vi "Clean FreeCache By Name.vi"(8 "error in (no error)":errorcluster, 10 "String":string, 11 "MDPtrMgr in":refnum<class "MDPtrMgr.lvclass">) -> (0 "error out":errorcluster, 3 "MDPtrMgr out":refnum<class "MDPtrMgr.lvclass">)   [LabVIEW 2017, in "MDPtr.lvlib" / "MDPtrMgr.lvclass"]
uses:
  MDPtrMgr.lvclass
  MDPtrMgr.lvclass/MDPtrMgr.ctl
  Factory/Def-MDPtrQ.ctl
  MDPtr TypeDef/MDPtr DataFrame-Memory.ctl
  MDPtr TypeDef/MDPtr DataFrame-Common.ctl
  <vilib>/Utility/Data Type/Type Definitions/Data Type.ctl
  <vilib>/Utility/Data Type/NI_Data Type.lvlib
  MDPtr.lvlib
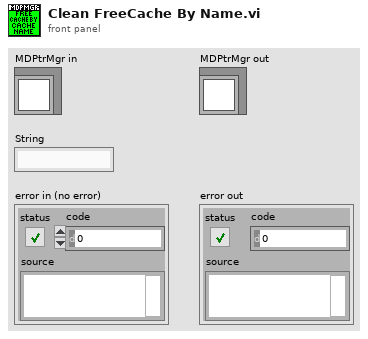
[diagram p1: front panel]
types:
  T1 = typedef "MDPtr.lvlib/MDPtrMgr.lvclass/Def-MDPtrQ.ctl" = refnum<queue>
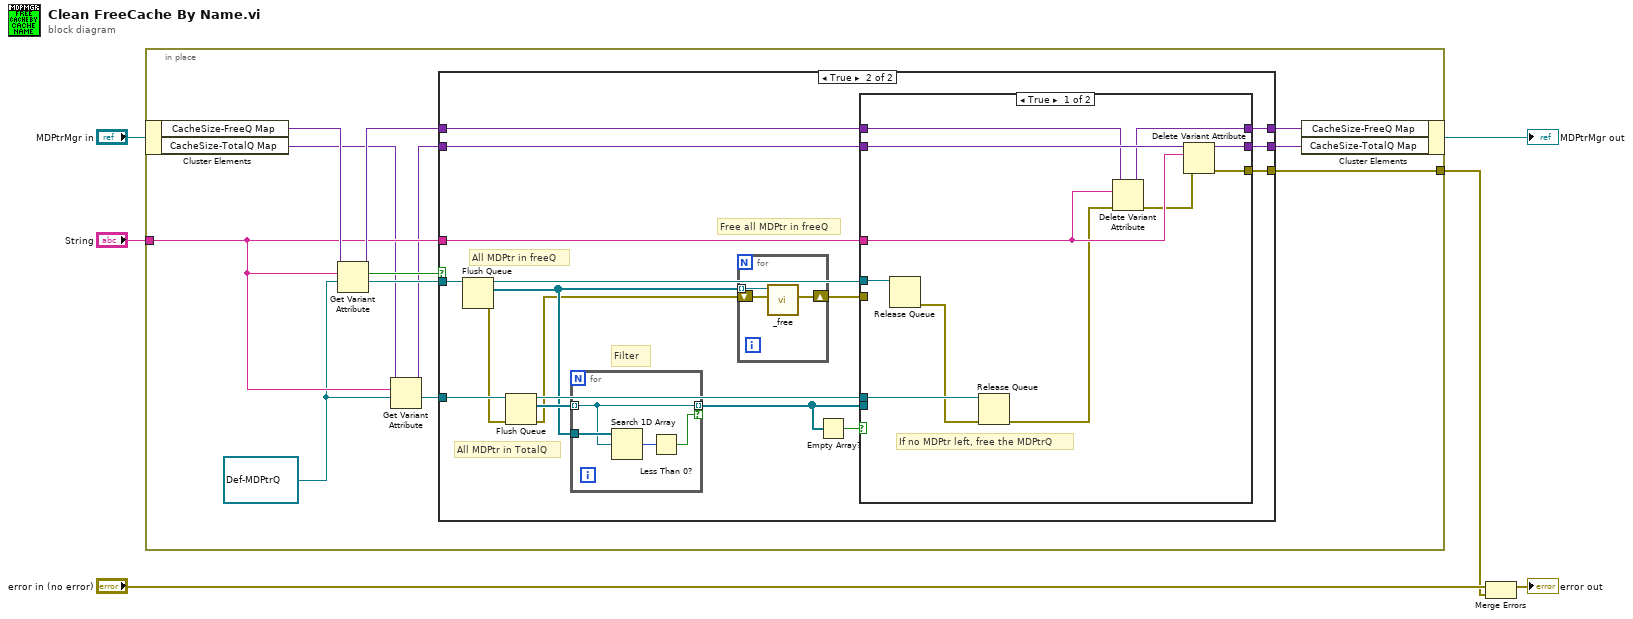
[diagram p0: block diagram]
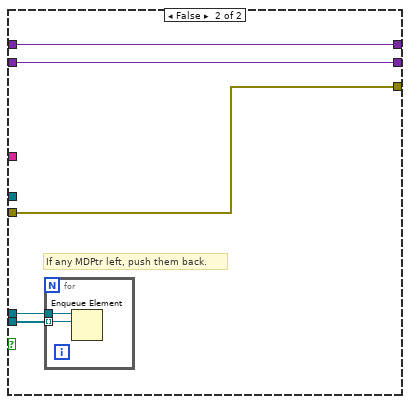
[diagram p3: hidden frame]
diagram:
  n1 = in-place "In Place Element Structure" {
    in-place-border: "String" -> [w12]
    in-place-border: [w7] -> w5
    w11 = T1 refnum ("MDPtrQueue")
    n2 = in-place-cluster #1("MDPtrMgr in") -> ("CacheSize-FreeQ Map"=w18:variant, "CacheSize-TotalQ Map"=w10:variant)
    n3 = Get Variant Attribute(Variant=w18, name=w12, default value (empty Variant)=w11) -> (duplicate Variant=w16:variant, found=w14:bool, value=w13:T1)  [unwired: 1 in, 1 out]
    n4 = Get Variant Attribute(Variant=w10, name=w12, default value (empty Variant)=w11) -> (duplicate Variant=w9:variant, value=w8:T1)  [unwired: 1 in, 2 out]
    n5 = case shown="True" w14 {
      tunnel: [w20 w37] -> w17
      tunnel: w9 -> [w20 w36]
      tunnel: w16 -> [w19 w35]
      tunnel: [w19 w34] -> w15
      tunnel: w12 -> [_ w33]
      tunnel: w13 -> [_ w31]
      tunnel: w8 -> [_ w30]
      tunnel: [_ w32] -> w7
      frame False {
      }
      frame True {
        # "Free all MDPtr in freeQ"
        # "Filter"
        # "All MDPtr in TotalQ"
        # "All MDPtr in freeQ"
        n6 = Flush Queue(queue=w31) -> (queue out=w24:T1, remaining elements=w25:refnum<data-value>[], error out=w23:errorcluster)  [unwired: 1 in]
        n7 = Flush Queue(queue=w30, error in (no error)=w23) -> (queue out=w28:T1, remaining elements=w29:refnum<data-value>[], error out=w22:errorcluster)
        n8 = for {
          tunnel: w29 -> [w60] mode=indexing
          tunnel: w25 -> [w62]
          tunnel: [w60] -> w27 mode=indexing if=w59
          n9 = Search 1D Array(1D array=w62, element=w60) -> (index of element=w61:i32)  [unwired: 1 in]
          n10 = Less Than 0?(x=w61) -> (x < 0?=w59:bool)
        }
        n11 = for {
          tunnel: w25 -> [w40] mode=indexing
          shift-right: [w38] -> w21
          shift-left: w22 -> [w39]
          n12 = call "_free.vi"("error in (no error)"=w39, "MDPtr DVR"=w40) -> ("error out"=w38:errorcluster)  [unwired: 8 in]
        }
        n13 = Empty Array?(array=w27) -> (empty?=w26:bool)
        n14 = case shown="True" w26 {
          tunnel: [w51 w56] -> w37
          tunnel: w36 -> [w50 w56]
          tunnel: w35 -> [w49 w55]
          tunnel: [w48 w55] -> w34
          tunnel: w33 -> [w47 _]
          tunnel: [w45 w52] -> w32
          tunnel: w28 -> [w44 w54]
          tunnel: w27 -> [_ w53]
          tunnel: w24 -> [w43 _]
          tunnel: w21 -> [_ w52]
          frame True {
            # "If no MDPtr left, free the MDPtrQ"
            n15 = Release Queue(queue=w43) -> (error out=w42:errorcluster)  [unwired: 2 in, 2 out]
            n16 = Release Queue(queue=w44, error in (no error)=w42) -> (error out=w41:errorcluster)  [unwired: 1 in, 2 out]
            n17 = Delete Variant Attribute(4:w41, 6:w47, 7:w49) -> (0:w46:errorcluster, 3:w48:variant)  [unwired: 1 out]
            n18 = Delete Variant Attribute(4:w46, 6:w47, 7:w50) -> (0:w45:errorcluster, 3:w51:variant)  [unwired: 1 out]
          }
          frame False {
            # "If any MDPtr left, push them back."
            n19 = for {
              tunnel: w53 -> [w57] mode=indexing
              tunnel: w54 -> [w58]
              n20 = Enqueue Element(queue=w58, element=w57) -> ()  [unwired: 2 in, 3 out]
            }
          }
        }
      }
    }
    n21 = in-place-cluster #1("CacheSize-FreeQ Map"=w15, "CacheSize-TotalQ Map"=w17) -> (→"MDPtrMgr out":refnum<class "MDPtrMgr.lvclass">)
  }
  n22 = Merge Errors("error in (no error)", w5) -> (→"error out":errorcluster)
